vi "mediaRobos_v2.vi"(8 "cameras array":dbl[](array[numeric]), 9 "grSim?":bool=TRUE, 10 "Field Size 2":T2, 11 "Array Robot Pose + CamID":T1(array[cluster])) -> (3 "Array":cluster{"x":dbl, "y":dbl, "robot_id":i32}[](array[cluster]))   [LabVIEW 2023]
panel:
  out "Array 2":u32[][](array[numeric])
  in  "Cam Intersection Widht":u32=6
  in  "Cam Intersection Lenght":u32=6
  in  "file path (use dialog) 2":path=path "C:/Users/RoboIme/git/sslview/Util/Farias2.csv"
  in  "cluster":cluster{"x":dbl, "y":dbl, "robot_id":i32}
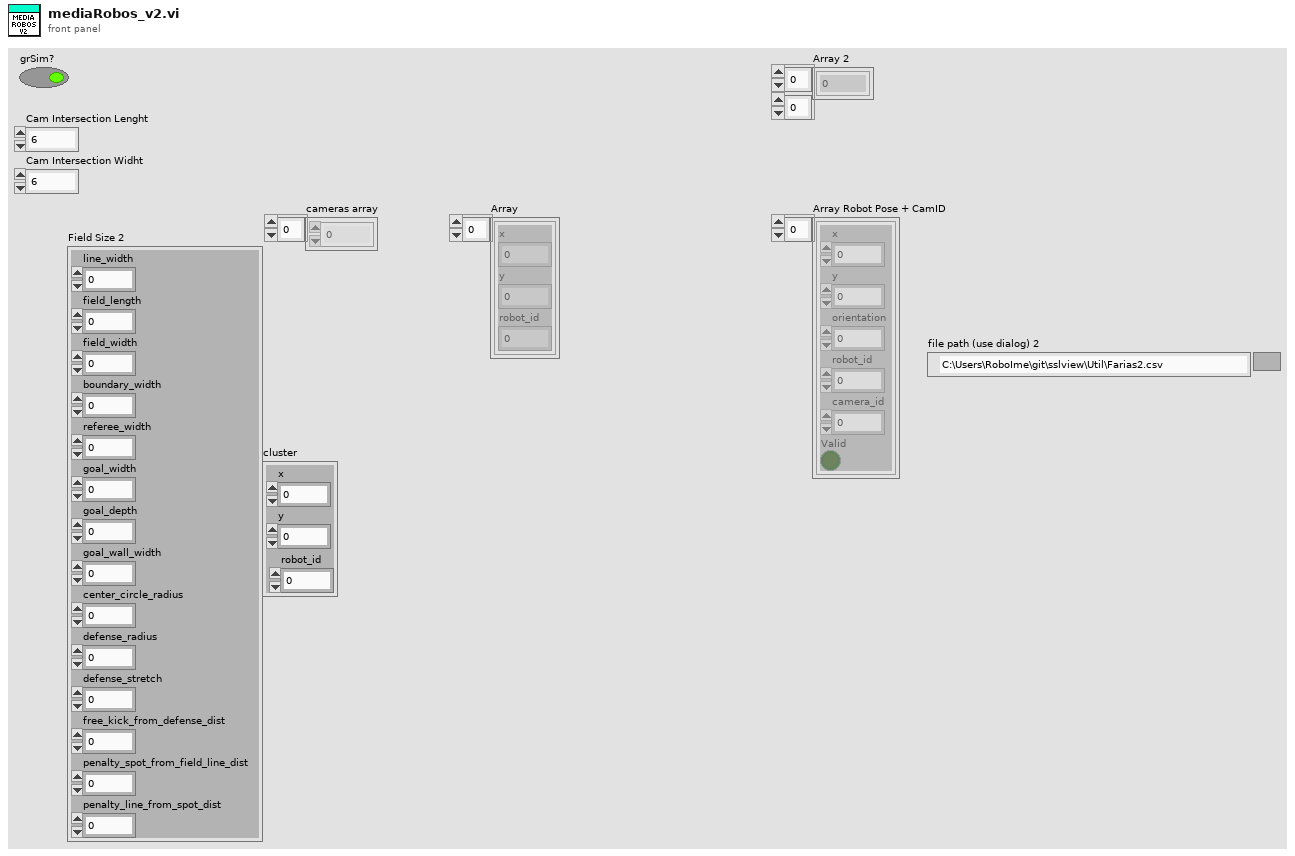
[diagram p1: front panel]
types:
  T1 = cluster{"x":sgl, "y":sgl, "orientation":sgl, "robot_id":u32, "camera_id":u32, "Valid":bool}[]
  T2 = cluster{"line_width":u32, "field_length":u32, "field_width":u32, "boundary_width":u32, "referee_width":u32, "goal_width":u32, "goal_depth":u32, "goal_wall_width":u32, "center_circle_radius":u32, "defense_radius":u32, "defense_stretch":u32, "free_kick_from_defense_dist":u32, "penalty_spot_from_field_line_dist":u32, "penalty_line_from_spot_dist":u32}
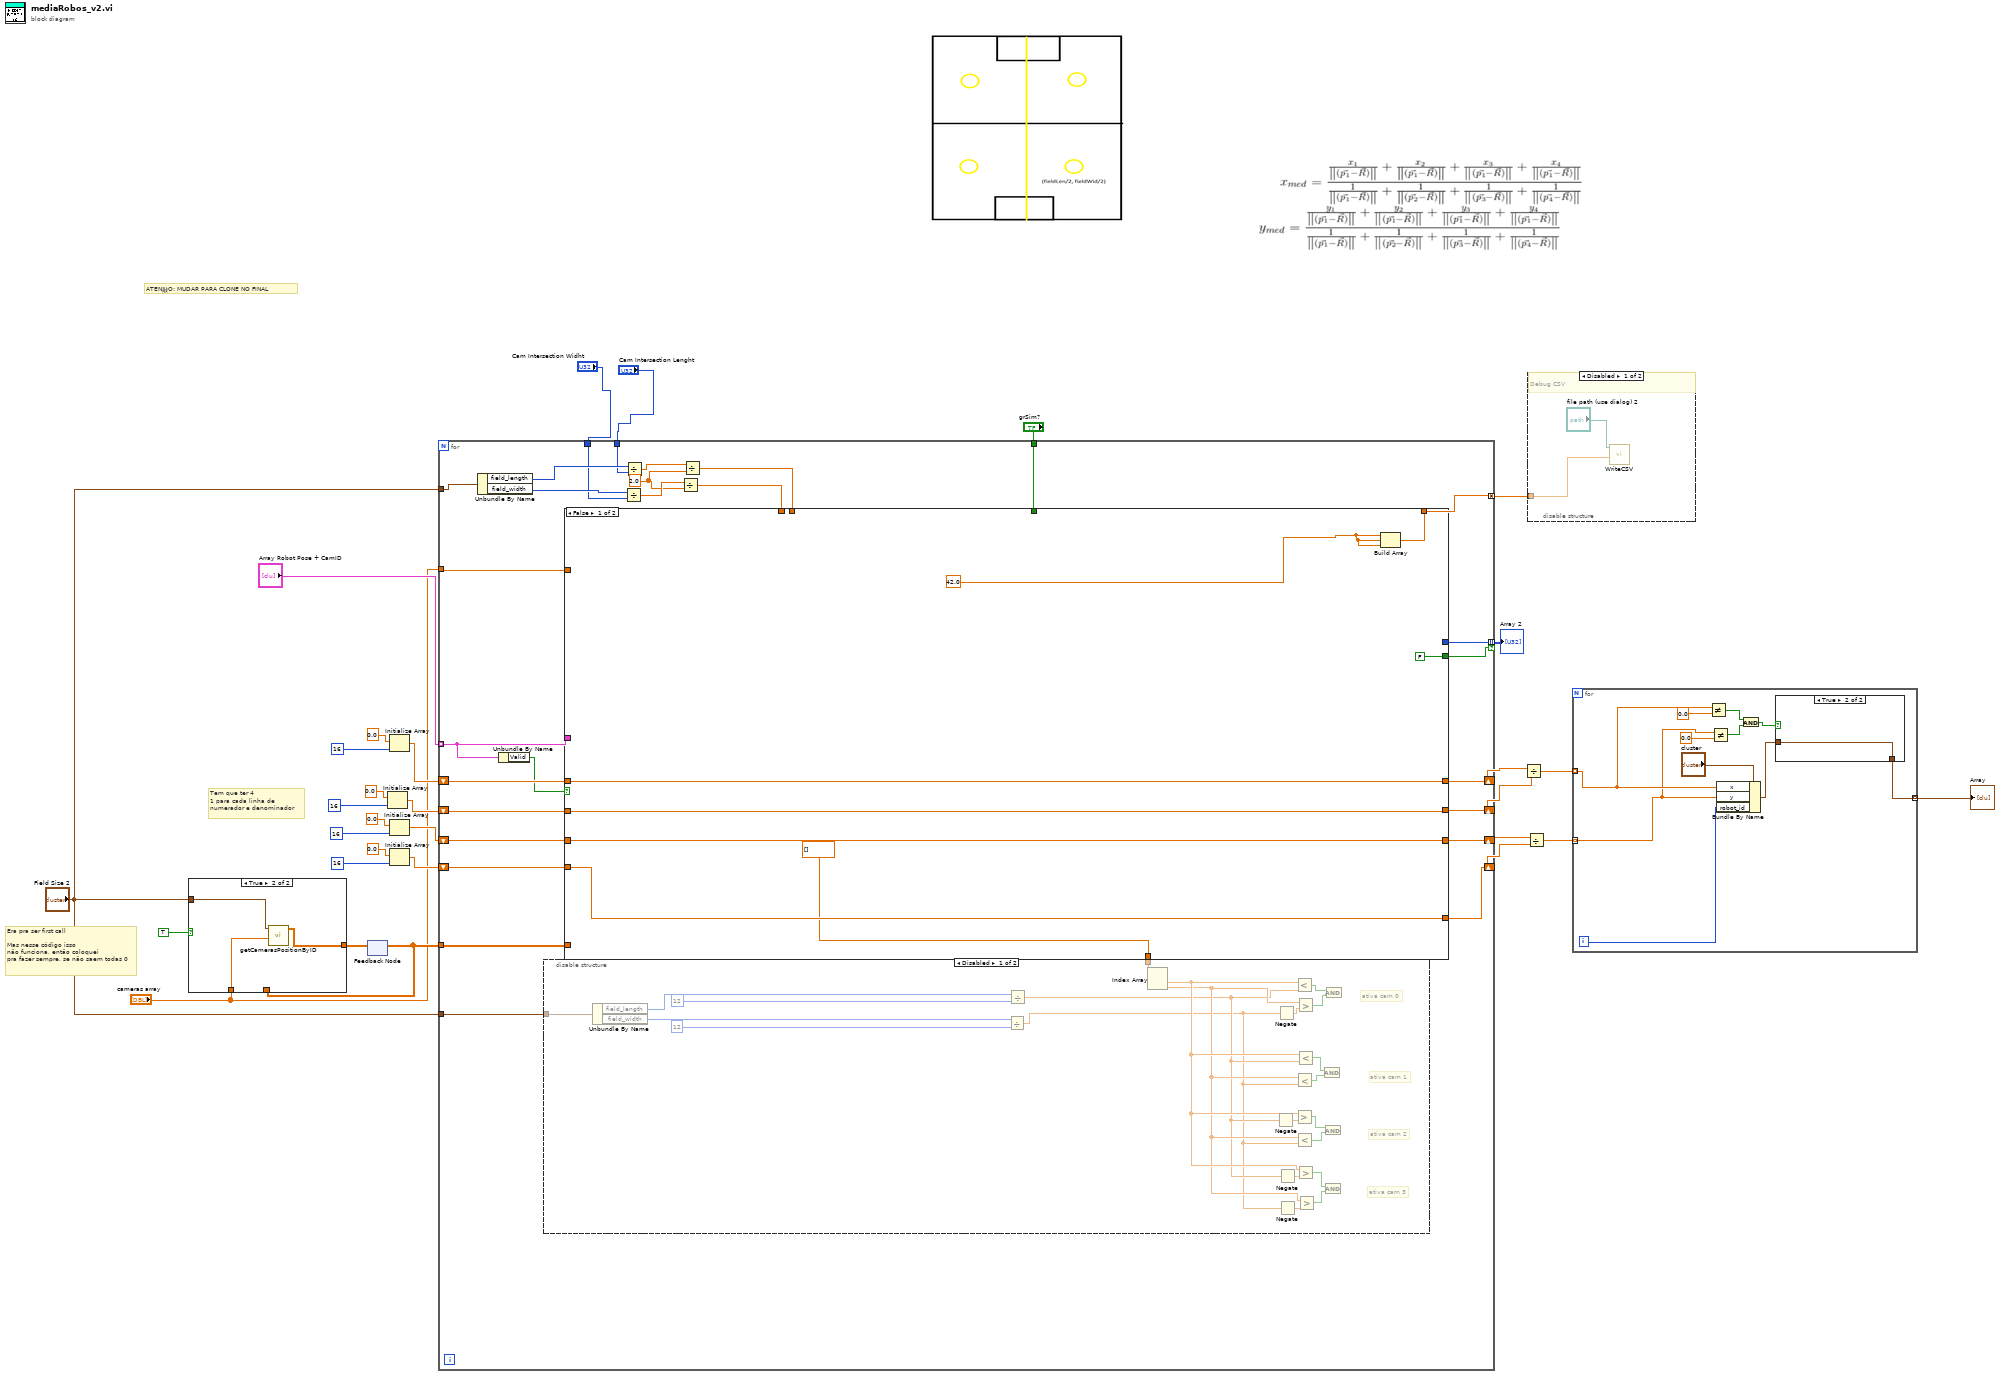
[diagram p0: block diagram]
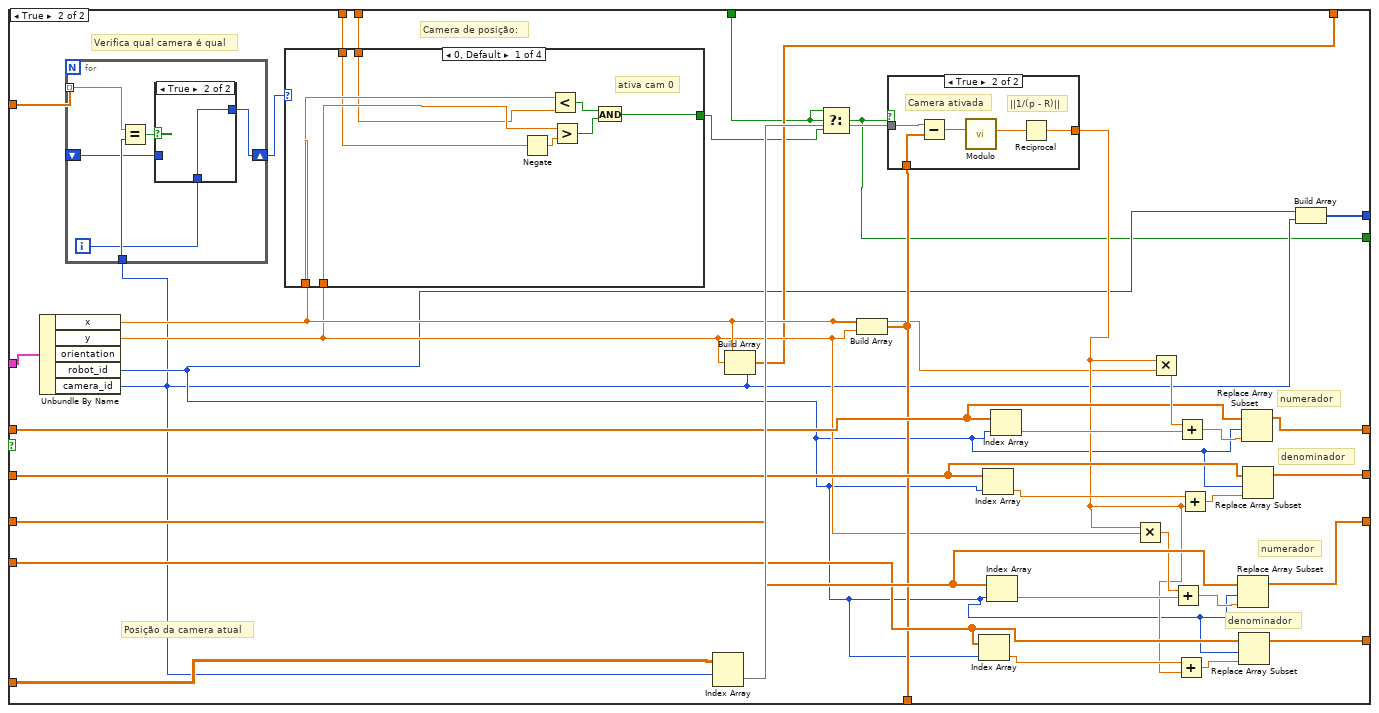
[diagram p4: hidden frame]
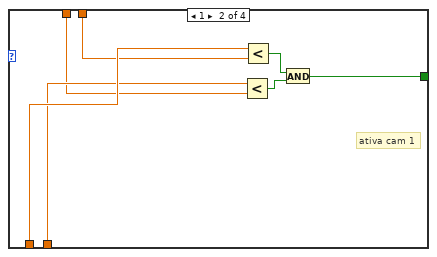
[diagram p5: hidden frame]
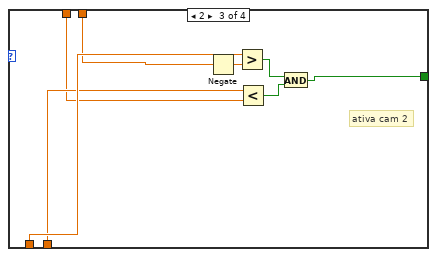
[diagram p6: hidden frame]
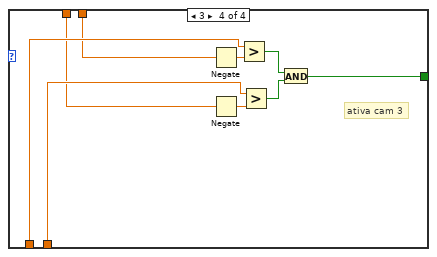
[diagram p7: hidden frame]
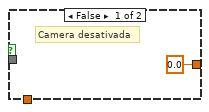
[diagram p9: hidden frame]
diagram:
  # "Era pra ser first call\n\nMas nesse código isso\nnão funciona, então coloquei\npra fazer sempre, se não saem todas 0"
  # "Tem que ter 4\n1 para cada linha de\nnumerador e denominador"
  # "ATEN敲O: MUDAR PARA CLONE NO FINAL"
  n1 = feedback #1() -> (w8:dbl[][])  [unwired: 1 in]
  n2 = case shown="True" TRUE {
    tunnel: "Field Size 2" -> [_ w34]
    tunnel: [w31 w33] -> w9
    tunnel: w8 -> [w31 _]
    tunnel: "cameras array" -> [_ w32]
    frame False {
    }
    frame True {
      n3 = call "getCamerasPositionByID.vi"("cameras id"=w32, "Field Size 2"=w34) -> ("Cameras Positions"=w33:dbl[][])  [unwired: 9 in]
    }
  }
  n4 = feedback-in #1(w9) -> ()
  n5 = Initialize Array(0.0 ("element"), 16 ("dimension size")) -> (w21:dbl[])
  n6 = Initialize Array(0.0 ("element"), 16 ("dimension size")) -> (w20:dbl[])
  n7 = Initialize Array(0.0 ("element"), 16 ("dimension size")) -> (w22:dbl[])
  n8 = Initialize Array(0.0 ("element"), 16 ("dimension size")) -> (w19:dbl[])
  n9 = for {
    tunnel: "Array Robot Pose + CamID" -> [w52] mode=indexing
    tunnel: w8 -> [w62]
    shift-right: [w61] -> w18
    shift-left: w22 -> [w55]
    shift-right: [w60] -> w17
    shift-left: w21 -> [w54]
    shift-right: [w59] -> w16
    shift-left: w20 -> [w57]
    shift-right: [w58] -> w15
    shift-left: w19 -> [w56]
    tunnel: [w53] -> w11 mode=concatenating
    tunnel: "Field Size 2" -> [w50]
    tunnel: "Field Size 2" -> [w48]
    tunnel: "Cam Intersection Lenght" -> [w45]
    tunnel: "Cam Intersection Widht" -> [w44]
    tunnel: "cameras array" -> [w43]
    tunnel: "grSim?" -> [w42]
    tunnel: [w41] -> w4 mode=indexing if=w35
    w38 = 2.0
    n10 = Unbundle By Name(w48) -> ("field_length"=w47:u32, "field_width"=w46:u32)
    n11 = Unbundle By Name(w52) -> ("Valid"=w51:bool)
    n12 = Divide(x=w46, y=w44) -> (x/y=w39:dbl)
    n13 = Divide(x=w47, y=w45) -> (x/y=w40:dbl)
    n14 = Divide(x=w39, y=w38) -> (x/y=w36:dbl)
    n15 = Divide(x=w40, y=w38) -> (x/y=w37:dbl)
    n16 = case shown="False" w51 {
      tunnel: w52 -> [_ w128]
      tunnel: w62 -> [_ w127]
      tunnel: [w92 w116] -> w61
      tunnel: [w91 w115] -> w60
      tunnel: [w90 w114] -> w59
      tunnel: [w89 w113] -> w58
      tunnel: w57 -> [w90 w112]
      tunnel: w56 -> [w89 w111]
      tunnel: w55 -> [w92 w110]
      tunnel: w54 -> [w91 w109]
      tunnel: [w88 w99] -> w53
      tunnel: [sgl[] [] w106] -> w49
      tunnel: w43 -> [_ w103]
      tunnel: w37 -> [_ w101]
      tunnel: w36 -> [_ w100]
      tunnel: w42 -> [_ w95]
      tunnel: [_ w96] -> w41
      tunnel: [FALSE w93] -> w35
      frame False {
        w87 = 42.0 ("element")
        n17 = Build Array(w87, w87, w87) -> (w88:dbl[])
      }
      frame True {
        # "Verifica qual camera é qual"
        # "Camera de posição:"
        # "denominador"
        # "numerador"
        # "denominador"
        # "numerador"
        # "Posição da camera atual"
        n18 = Unbundle By Name(w128) -> ("x"=w105:sgl, "y"=w104:sgl, "robot_id"=w98:u32, "camera_id"=w97:u32)  [unwired: 1 out]
        n19 = for {
          tunnel: w103 -> [w165] mode=indexing
          tunnel: w97 -> [w166]
          shift-right: [w162] -> w102
          shift-left: _ -> [w161]
          i -> [w163]
          n20 = Equal?(x=w165, y=w166) -> (x = y?=w164:bool)
          n21 = case shown="True" w164 {
            tunnel: w163 -> [_ w168]
            tunnel: [w167 w168] -> w162
            tunnel: w161 -> [w167 _]
            frame False {
            }
            frame True {
            }
          }
        }
        n22 = case shown="0, Default" w102 {
          tunnel: w105 -> [w133 w141 w148 w156]
          tunnel: w104 -> [w132 w140 w147 w155]
          tunnel: [w129 w137 w144 w152] -> w94
          tunnel: w101 -> [w131 w139 w146 w154]
          tunnel: w100 -> [w130 w138 w145 w153]
          frame 0, Default {
            # "ativa cam 0"
            n23 = Negate(x=w130) -> (-x=w134:dbl)
            n24 = Less?(x=w133, y=w131) -> (x < y?=w136:bool)
            n25 = Greater?(x=w132, y=w134) -> (0:w135:bool)
            n26 = And(x=w136, y=w135) -> (x .and. y?=w129:bool)
          }
          frame 1 {
            # "ativa cam 1"
            n27 = Less?(x=w140, y=w138) -> (x < y?=w143:bool)
            n28 = Less?(x=w141, y=w139) -> (x < y?=w142:bool)
            n29 = And(x=w142, y=w143) -> (x .and. y?=w137:bool)
          }
          frame 2 {
            # "ativa cam 2"
            n30 = Negate(x=w146) -> (-x=w151:dbl)
            n31 = Greater?(x=w148, y=w151) -> (0:w150:bool)
            n32 = Less?(x=w147, y=w145) -> (x < y?=w149:bool)
            n33 = And(x=w150, y=w149) -> (x .and. y?=w144:bool)
          }
          frame 3 {
            # "ativa cam 3"
            n34 = Negate(x=w154) -> (-x=w160:dbl)
            n35 = Negate(x=w153) -> (-x=w159:dbl)
            n36 = Greater?(x=w156, y=w160) -> (0:w157:bool)
            n37 = Greater?(x=w155, y=w159) -> (0:w158:bool)
            n38 = And(x=w157, y=w158) -> (x .and. y?=w152:bool)
          }
        }
        n39 = Index Array(array=w127, index (row)=w97) -> (element=w121:dbl[])  [unwired: 1 in]
        n40 = Build Array(w105, w104, w97) -> (w99:sgl[])
        n41 = Select(t=w95, s=w95, f=w94) -> (s? t:f=w93:bool)
        n42 = Build Array(w105, w104) -> (w106:sgl[])
        n43 = case shown="True" w93 {
          tunnel: w121 -> [_ w172]
          tunnel: [0.0 w171] -> w107
          tunnel: w106 -> [_ w170]
          frame False {
            # "Camera desativada"
          }
          frame True {
            # "Camera ativada"
            # "||1/(p - R)||"
            n44 = Subtract(x=w172, y=w170) -> (x-y=w174:dbl[])
            n45 = call "Modulo.vi"("2D vector"=w174) -> ("Modulo"=w173:dbl)  [unwired: 10 in]
            n46 = Reciprocal(x=w173) -> (1/x=w171:dbl)
          }
        }
        n47 = Index Array(array=w111, index=w98) -> (element=w117:dbl)
        n48 = Index Array(array=w109, index=w98) -> (element=w119:dbl)
        n49 = Index Array(array=w112, index=w98) -> (element=w118:dbl)
        n50 = Index Array(array=w110, index=w98) -> (element=w120:dbl)
        n51 = Multiply(x=w107, y=w104) -> (x*y=w108:dbl)
        n52 = Multiply(x=w107, y=w105) -> (x*y=w126:dbl)
        n53 = Add(x=w108, y=w118) -> (x+y=w123:dbl)
        n54 = Add(x=w117, y=w107) -> (x+y=w122:dbl)
        n55 = Add(x=w126, y=w120) -> (x+y=w125:dbl)
        n56 = Add(x=w119, y=w107) -> (x+y=w124:dbl)
        n57 = Replace Array Subset(array=w112, new element=w123, index=w98) -> (w114:dbl[])
        n58 = Replace Array Subset(array=w111, new element=w122, index=w98) -> (w113:dbl[])
        n59 = Replace Array Subset(array=w110, new element=w125, index=w98) -> (w116:dbl[])
        n60 = Replace Array Subset(array=w109, new element=w124, index=w98) -> (w115:dbl[])
        n61 = Build Array(w98, w97) -> (w96:u32[])
      }
    }
    n62 = disable-structure shown="Disabled" {
      disable-tunnel: w50 -> [w84 _]
      disable-tunnel: w49 -> [w79 _]
      frame Disabled {
        # "ativa cam 3"
        # "ativa cam 2"
        # "ativa cam 1"
        # "ativa cam 0"
        n63 = Unbundle By Name(w84) -> ("field_length"=w80:u32, "field_width"=w81:u32)
        n64 = Divide(x=w81, y=u32 12) -> (x/y=w63:dbl)
        n65 = Divide(x=w80, y=u32 12) -> (x/y=w64:dbl)
        n66 = Index Array(array=w79) -> (element #1=w66:sgl, element #2=w65:sgl)  [unwired: 2 in]
        n67 = Negate(x=w64) -> (-x=w73:dbl)
        n68 = Negate(x=w63) -> (-x=w76:dbl)
        n69 = Negate(x=w64) -> (-x=w70:dbl)
        n70 = Negate(x=w63) -> (-x=w69:dbl)
        n71 = Less?(x=w66, y=w64) -> (x < y?=w78:bool)
        n72 = Greater?(x=w66, y=w73) -> (0:w72:bool)
        n73 = Less?(x=w65, y=w63) -> (x < y?=w75:bool)
        n74 = Less?(x=w65, y=w63) -> (x < y?=w71:bool)
        n75 = Greater?(x=w65, y=w76) -> (0:w77:bool)
        n76 = Less?(x=w66, y=w64) -> (x < y?=w74:bool)
        n77 = Greater?(x=w66, y=w70) -> (0:w67:bool)
        n78 = Greater?(x=w65, y=w69) -> (0:w68:bool)
        n79 = And(x=w74, y=w75) -> ()  [unwired: 1 out]
        n80 = And(x=w72, y=w71) -> ()  [unwired: 1 out]
        n81 = And(x=w67, y=w68) -> ()  [unwired: 1 out]
        n82 = And(x=w78, y=w77) -> ()  [unwired: 1 out]
      }
      frame Enabled {
      }
    }
  }
  "Array 2" <- w4
  n83 = Divide(x=w18, y=w17) -> (x/y=w14:dbl[])
  n84 = Divide(x=w16, y=w15) -> (x/y=w13:dbl[])
  n85 = disable-structure "Diagram Disable Structure" shown="Disabled" {
    disable-tunnel: w11 -> [w176 _]
    frame Disabled {
      # "Debug CSV"
      n86 = call "WriteCSV.vi"("array"=w176, "file path (use dialog)"="file path (use dialog) 2") -> ()  [unwired: 10 in]
    }
    frame Enabled {
    }
  }
  n87 = for {
    tunnel: w14 -> [w186] mode=indexing
    tunnel: w13 -> [w183] mode=indexing
    tunnel: [w179] -> w12 mode=indexing
    i -> [w187]
    n88 = Not Equal?(x=w186, y=0.0) -> (x != y?=w182:bool)
    n89 = Not Equal?(x=w183, y=0.0) -> (x != y?=w181:bool)
    n90 = Bundle By Name(cluster="cluster", "x"=w186, "y"=w183, "robot_id"=w187) -> (w178:cluster{"x":dbl, "y":dbl, "robot_id":i32})
    n91 = And(x=w182, y=w181) -> (x .and. y?=w180:bool)
    n92 = case shown="True" w180 {
      tunnel: [w188 w189] -> w179
      tunnel: w178 -> [w188 w189]
      frame False {
      }
      frame True {
      }
    }
  }
  "Array" <- w12
